vi "Make_Settings_Item.vi"(8 "error in (no error)":errorcluster, 10 "address":string[](array[string]), 11 "userFolder in":refnum<class "userFolder.lvclass">) -> (0 "error out":errorcluster, 3 "IB_Settings_Item.lvclass":refnum<class "IB_Settings_Item.lvclass">)   [LabVIEW 2020, in "userFolder.lvclass"]
uses:
  <vilib>/AppBuilder/IB_Classes/Destination/userFolder/userFolder.lvclass
  <vilib>/AppBuilder/IB_Classes/Destination/userFolder/userFolder.lvclass/userFolder.ctl
  <vilib>/AppBuilder/IB_Classes/Settings_Item_Destination/IB_Settings_Item_Destination.lvclass
  <vilib>/AppBuilder/IB_Classes/Settings_Item/IB_Settings_Item.lvclass
  e:/builds/penguin/labview/branches/2020/dev/dist/vi.lib/AppBuilder/IB_Classes/Settings_Item/IB_Settings_Item.lvclass
  e:/builds/penguin/labview/branches/2020/dev/dist/vi.lib/AppBuilder/IB_Classes/Settings_Item_Destination/IB_Settings_Item_Destination.lvclass
  e:/builds/penguin/labview/branches/2020/dev/dist/vi.lib/AppBuilder/IB_Classes/Destination/IB_Destination.lvclass
  e:/builds/penguin/labview/branches/2020/dev/dist/vi.lib/AppBuilder/IB_Classes/Destination/userFolder/userFolder.lvclass
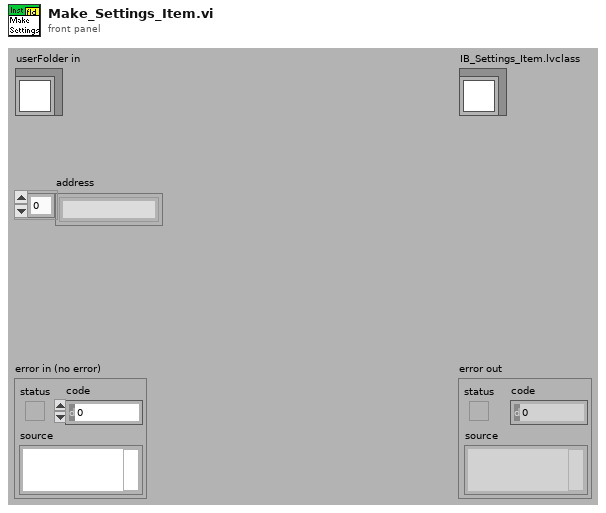
[diagram p1: front panel]
types:
  T1 = typedef "IB_Settings_Item.ctl" = cluster{"address":string[], "Attributes":i16, "RegCOM":bool, "unlock":bool}
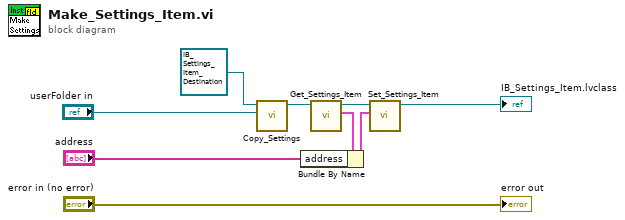
[diagram p0: block diagram]
diagram:
  n1 = call-dynamic "Copy_Settings.vi"("LabVIEW Object"="userFolder in", "IB_Settings_Item_Destination in"=refnum<class "IB_Settings_Item_Destination.lvclass"> refnum ("IB_Settings_Item_Destination.lvclass")) -> ("IB_Settings_Item_Destination out"=w7:refnum<class "IB_Settings_Item_Destination.lvclass">)  [unwired: 8 in, 1 out]
  n2 = call <vilib>:"Get_Settings_Item.vi"("IB_Settings_Item in"=w7) -> ("data"=w6:T1, "IB_Settings_Item out"=w8:refnum<class "IB_Settings_Item_Destination.lvclass">)  [unwired: 8 in, 1 out]
  n3 = Bundle By Name(cluster=w6, "address"="address") -> (w5:T1)
  n4 = call <vilib>:"Set_Settings_Item.vi"("data"=w5, "IB_Settings_Item in"=w8) -> ("IB_Settings_Item out"=→"IB_Settings_Item.lvclass":refnum<class "IB_Settings_Item_Destination.lvclass">)  [unwired: 8 in, 1 out]
  "error out" <- "error in (no error)"
